vi "gun_turret_man_ovr.vi"(9 "Overide":dbl, 10 "gun_rt_slow_downstream_data out in":T1, 11 "Trigger Vision":bool) -> (3 "gun_rt_slow_downstream_data out out":T1)   [LabVIEW 2011]
uses:
  gun_rt_slow_downstream_data.ctl
  2012vision/Camera State.ctl
panel:
  in  "man_scale":dbl=0.3
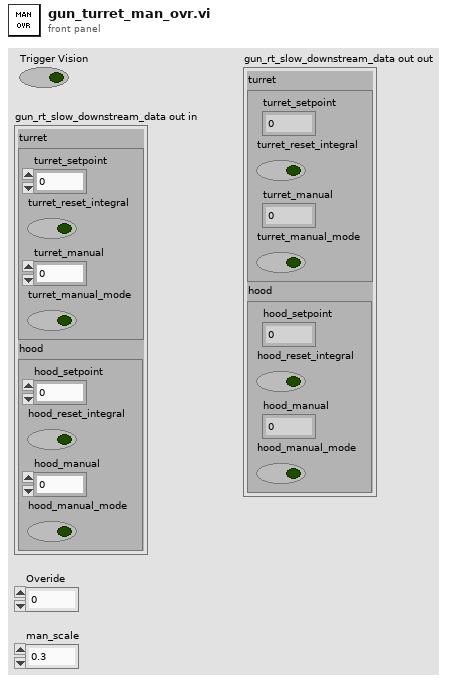
[diagram p1: front panel]
types:
  T1 = typedef "gun_rt_slow_downstream_data.ctl" = cluster{"turret":cluster{"turret_setpoint":dbl, "turret_reset_integral":bool, "turret_manual":dbl, "turret_manual_mode":bool}, "hood":cluster{"hood_setpoint":dbl, "hood_reset_integral":bool, "hood_manual":dbl, "hood_manual_mode":bool}}
  T2 = typedef "Camera State.ctl" = enum16{"No Targets", "Low Confidence", "Medium Confidence", "High Confidence", "Camera Error"}
  T3 = enum16{"Get Latest Data", "Get Local Data", "Get Remote Data", "Set Local Data", "Set Remote Data"}
  T4 = cluster{"X Position":dbl, "Distance":dbl, "Camera State":T2}
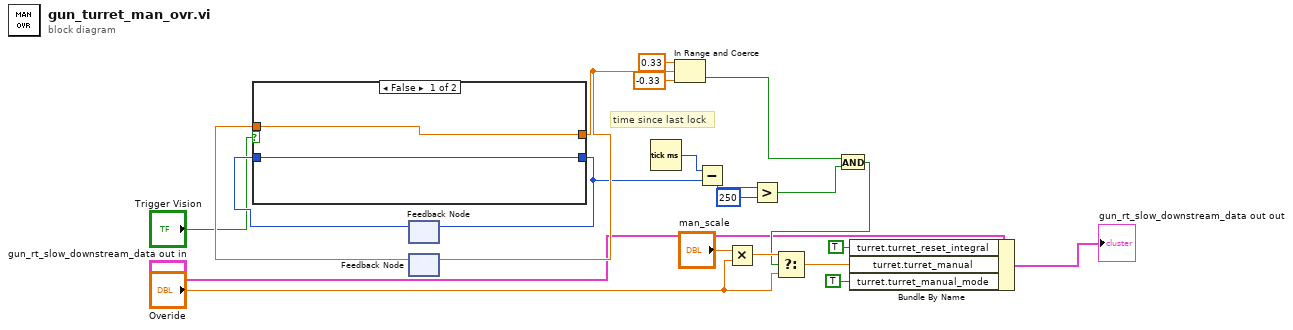
[diagram p0: block diagram]
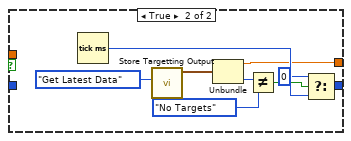
[diagram p2: hidden frame]
diagram:
  # "time since last lock"
  n1 = feedback #1() -> (w6:u32)  [unwired: 1 in]
  n2 = feedback #2() -> (w14:dbl)  [unwired: 1 in]
  n3 = case shown="False" "Trigger Vision" {
    tunnel: [w23 w25] -> w8
    tunnel: w6 -> [w23 _]
    tunnel: [w22 w24] -> w15
    tunnel: w14 -> [w22 _]
    frame False {
    }
    frame True {
      n4 = Tick Count (ms)() -> (millisecond timer value=w27:u32)
      n5 = call "Store Targetting Output.vi"("mode"=T3."Get Latest Data") -> ("Targetting Output"=w31:T4)  [unwired: 10 in]
      n6 = Unbundle(w31) -> ("X Position"=w24:dbl, "Camera State"=w30:T2)  [unwired: 1 out]
      n7 = Not Equal?(x=w30, y=Camera_State."No Targets") -> (x != y?=w28:bool)
      n8 = Select(t=u32 0, s=w28, f=w27) -> (s? t:f=w25:u32)
    }
  }
  n9 = feedback-in #1(w8) -> ()
  n10 = feedback-in #2(w15) -> ()
  n11 = Tick Count (ms)() -> (millisecond timer value=w7:u32)
  n12 = In Range and Coerce(upper limit=0.33, x=w15, lower limit=-0.33) -> (In Range?=w18:bool)  [unwired: 1 out]
  n13 = Subtract(x=w7, y=w8) -> (x-y=w9:u32)
  n14 = Multiply(x="man_scale", y="Overide") -> (x*y=w19:dbl)
  n15 = Greater?(x=w9, y=u32 250) -> (0:w11:bool)
  n16 = And(x=w18, y=w11) -> (x .and. y?=w13:bool)
  n17 = Select(t=w19, s=w13, f="Overide") -> (s? t:f=w12:dbl)
  n18 = Bundle By Name(cluster="gun_rt_slow_downstream_data out in", "turret.turret_reset_integral"=TRUE, "turret.turret_manual"=w12, "turret.turret_manual_mode"=TRUE) -> (→"gun_rt_slow_downstream_data out out":T1)
